vi "FTW-JSON-Native-HandleUnflattenErrors.vi"(7 "error in":errorcluster) -> (8 "error out":errorcluster)   [LabVIEW 2015]
uses:
  Error/FTW-ERR-Clear.vi
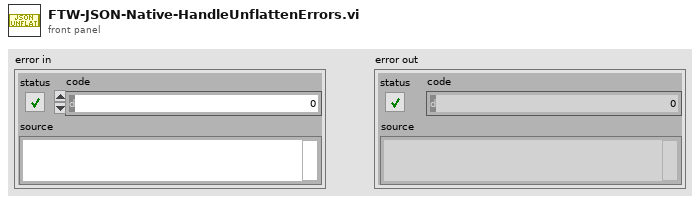
[diagram p1: front panel]
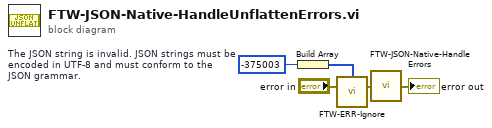
[diagram p0: block diagram]
diagram:
  w2 = -375003  # The JSON string is invalid. JSON strings must be encoded in UTF-8 and must conform to the JSON grammar.
  n1 = Build Array(w2) -> (w3:i32[])
  n2 = call "FTW-ERR-Ignore.vi"("Codes to filter"=w3, "error to filter"="error in") -> ("filtered error"=w4:errorcluster)  [unwired: 13 in]
  n3 = call "FTW-JSON-Native-HandleErrors.vi"("error in"=w4) -> ("error out"=→"error out":errorcluster)  [unwired: 14 in]
